vi "FP time to string.vi"() -> (0 "time string":string)   [LabVIEW 2014]
doc: "This VI converts the present time to a string followed by a carriage return."
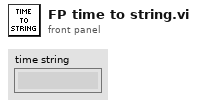
[diagram p1: front panel]
types:
  T1 = typedef "LVDateTimeRec.ctl" = cluster{"fractional second":dbl, "second":i32, "minute":i32, "hour":i32, "day of month":i32, "month":i32, "year":i32, "day of week":i32, "day of year":i32, "DST":i32}
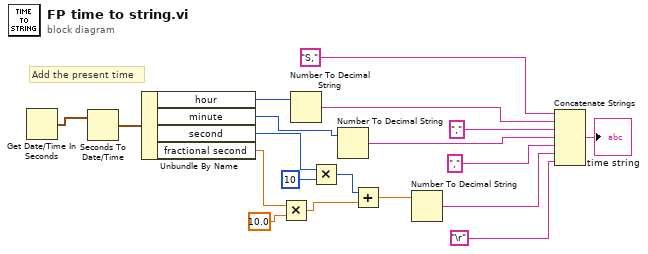
[diagram p0: block diagram]
diagram:
  # "Add the present time"
  n1 = Get Date/Time In Seconds() -> (seconds since 1Jan1904=w18:timestamp)
  n2 = Seconds To Date/Time(time stamp (now)=w18) -> (date time rec=w17:T1)  [unwired: 1 in]
  n3 = Unbundle By Name(w17) -> ("hour"=w16:i32, "minute"=w15:i32, "second"=w7:i32, "fractional second"=w9:dbl)
  n4 = Multiply(x=w9, y=10.0) -> (x*y=w4:dbl)
  n5 = Number To Decimal String(number=w16) -> (decimal integer string=w14:string)  [unwired: 1 in]
  n6 = Multiply(x=w7, y=10) -> (x*y=w5:i32)
  n7 = Number To Decimal String(number=w15) -> (decimal integer string=w13:string)  [unwired: 1 in]
  n8 = Add(x=w5, y=w4) -> (x+y=w3:dbl)
  n9 = Number To Decimal String(number=w3) -> (decimal integer string=w12:string)  [unwired: 1 in]
  n10 = Concatenate Strings("S,", w14, "," ("string"), w13, "," ("string"), w12, "\r") -> (→"time string":string)
